vi "SOLAR PLANT MONITORING SYSTEM IN LabVIEW 2.vi"() -> ()   [LabVIEW 2025]
uses:
  <vilib>/Utility/error.llb/DialogType.ctl
  <vilib>/DAQmx/read.llb/DAQmx Read (Analog DBL 1Chan 1Samp).vi
  <vilib>/DAQmx/create/channels.llb/DAQmx Create Channel (AI-Voltage-Basic).vi
  <vilib>/DAQmx/miscellaneous.llb/DAQmx Fill In Error Info.vi
panel:
  in  "custom scale name":tag
  out "I-V curve":cluster{"Y":dbl[], "Y":dbl[]}[](graph)
  out "P-V curve":cluster{"Y":dbl[], "Y":dbl[]}[](graph)
  out "Power curve":dbl(graph)
  out "POWER":dbl(knob) scale=0.0..10.0
  out "Current Chart":dbl(graph)
  out "?":dbl(knob) scale=0.0..10.0
  out "Voltage Chart":dbl(graph)
  out "?":dbl(knob) scale=0.0..50.0
  in  "units":i32(ring)=10348 items=["Volts"=10348, "From Custom Scale"=10065]
  in  "physical channels":tag
  in  "stop":bool
  # "VOLTAGE SENSOR"
  # "CURRENT SENSOR"
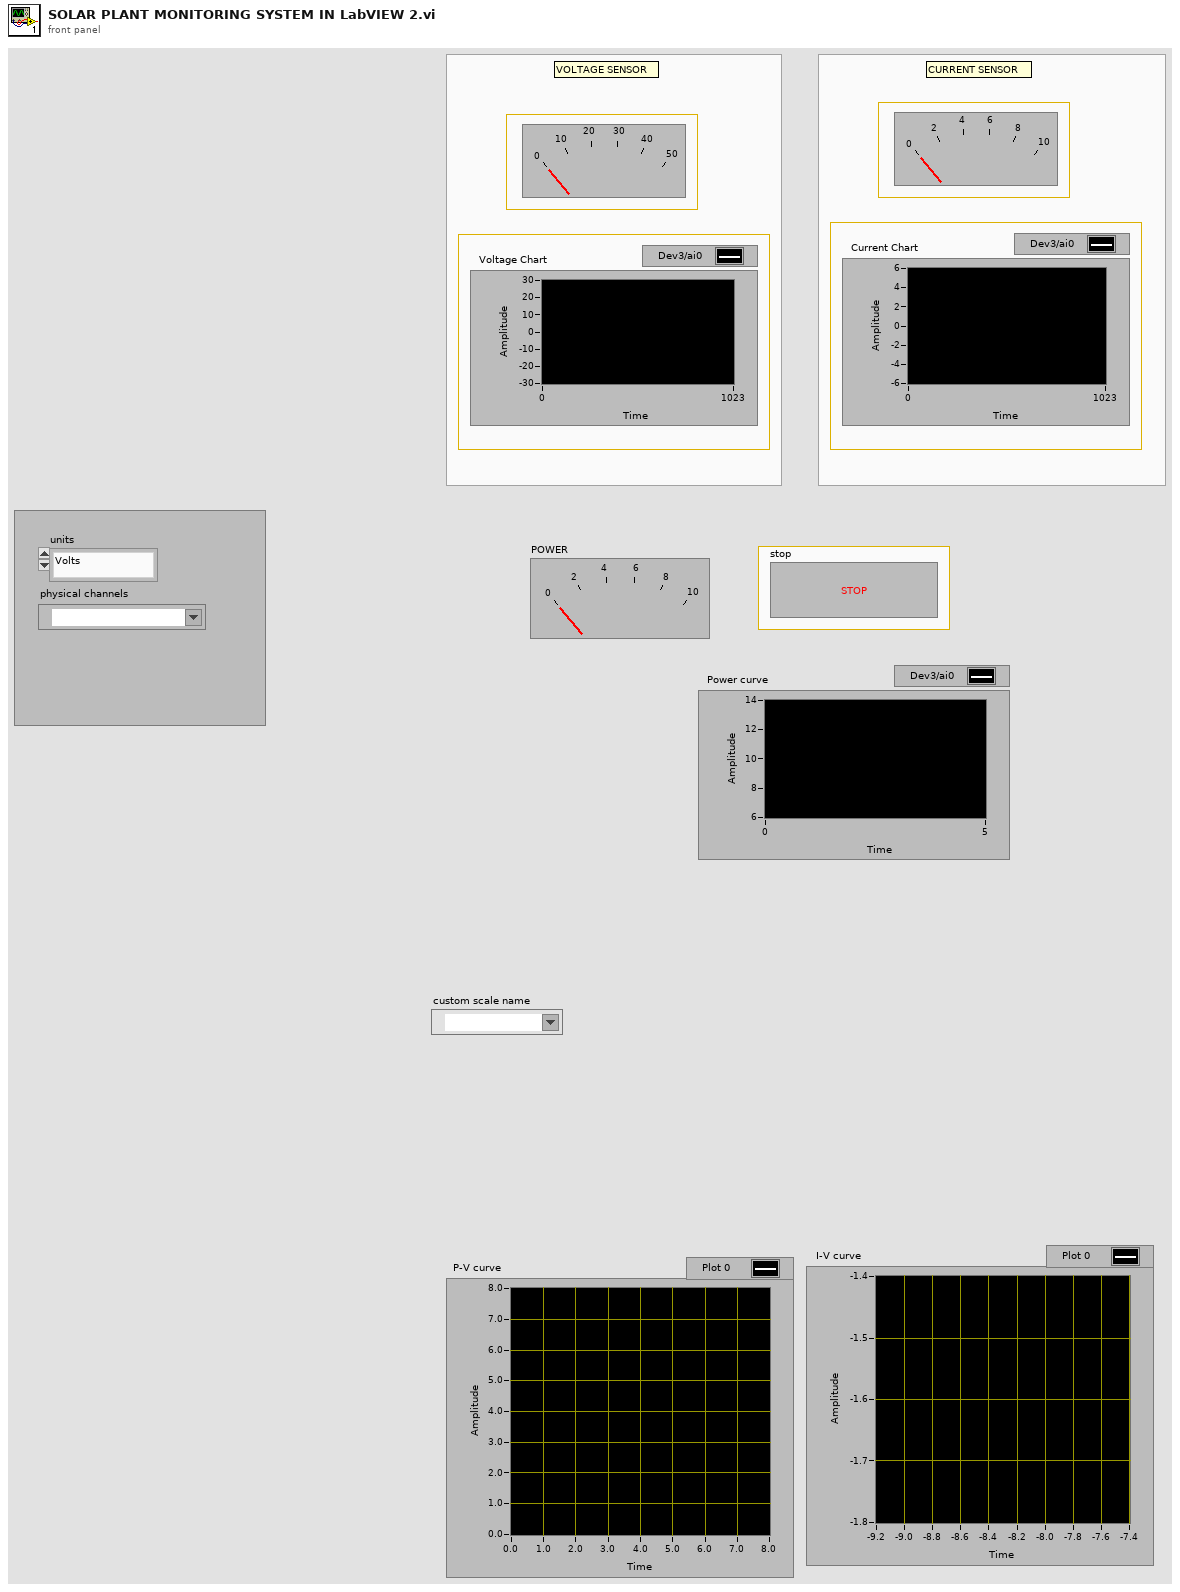
[diagram p1: front panel]
types:
  T1 = typedef "DialogType.ctl" = u16
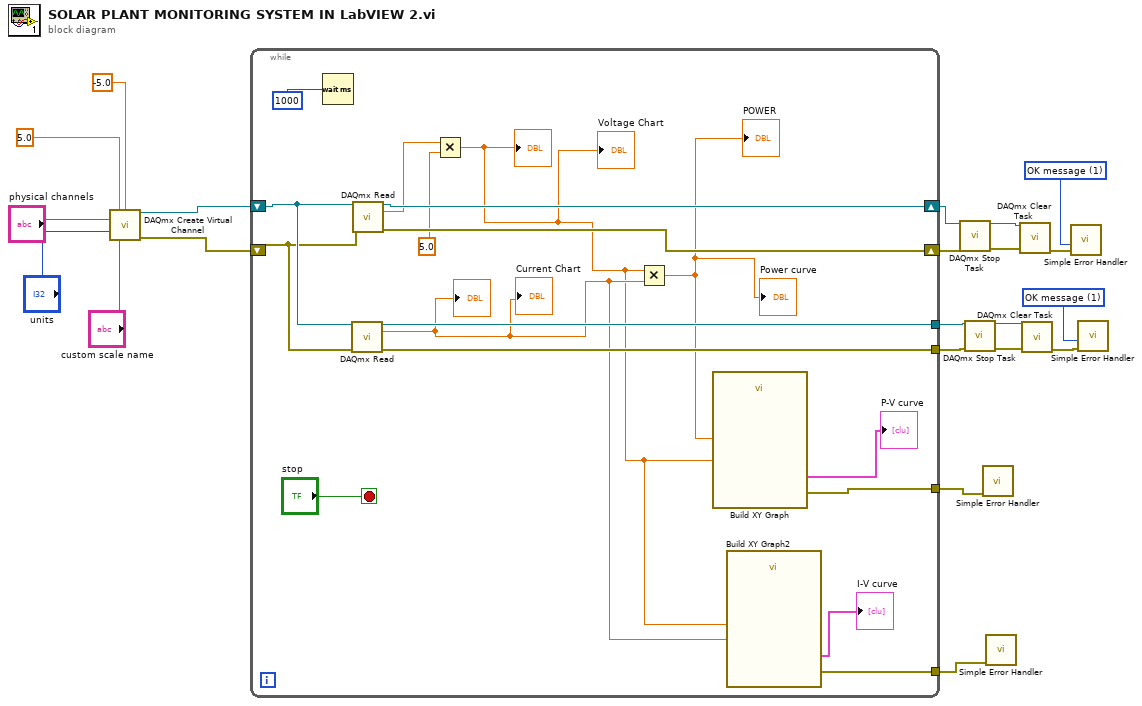
[diagram p0: block diagram]
diagram:
  w8 = T1 1 items=["no dialog", "OK message", "continue or stop message", "OK message + warnings", "continue/stop + warnings"] ("type of dialog (OK msg:1)")
  w12 = T1 1 items=["no dialog", "OK message", "continue or stop message", "OK message + warnings", "continue/stop + warnings"] ("type of dialog (OK msg:1)")
  n1 = call-poly <vilib>:"DAQmx Create Virtual Channel.vi"("maximum value"=5.0, "minimum value"=-5.0, "physical channels"="physical channels", "units"="units", "custom scale name"="custom scale name") -> ("task out"=w19:refnum<k21>, "error out"=w18:errorcluster)  [unwired: 9 in]
  n2 = while {
    shift-right: [w37] -> w16
    shift-left: w19 -> [w33]
    shift-right: [w36] -> w17
    shift-left: w18 -> [w32]
    tunnel: [w31] -> w7
    tunnel: [w30] -> w6
    tunnel: [w27] -> w5
    tunnel: [w22] -> w2
    stop <- "stop" stop-if-true
    n3 = Wait (ms)(milliseconds to wait=u32 1000) -> ()  [unwired: 1 out]
    n4 = call-poly <vilib>:"DAQmx Read.vi"("task/channels in"=w33, "error in"=w32) -> ("task out"=w31:refnum<k21>, "data"=w24:dbl, "error out"=w30:errorcluster)  [unwired: 11 in]
    "?" <- w24
    "Current Chart" <- w24
    n5 = call-poly <vilib>:"DAQmx Read.vi"("task/channels in"=w33, "error in"=w32) -> ("task out"=w37:refnum<k21>, "data"=w35:dbl, "error out"=w36:errorcluster)  [unwired: 11 in]
    n6 = Multiply(x=w35, y=5.0) -> (x*y=w23:dbl)
    "?" <- w23
    "Voltage Chart" <- w23
    n7 = Multiply(x=w23, y=w24) -> (x*y=w28:dbl)
    "POWER" <- w28
    "Power curve" <- w28
    n8 = call "Build XY Graph"("Y Input"=w23, "X Input"=w28) -> ("error out"=w27:errorcluster, "XY Graph"=→"P-V curve":cluster{"X":dbl[], "Y":dbl[]}[])  [unwired: 8 in]
    n9 = call "Build XY Graph2"("Y Input"=w24, "X Input"=w23) -> ("error out"=w22:errorcluster, "XY Graph"=→"I-V curve":cluster{"X":dbl[], "Y":dbl[]}[])  [unwired: 8 in]
  }
  n10 = call <vilib>:"DAQmx Stop Task.vi"("task/channels in"=w16, "error in"=w17) -> ("task out"=w15:refnum<k21>, "error out"=w14:errorcluster)  [unwired: 12 in]
  n11 = call <vilib>:"DAQmx Stop Task.vi"("task/channels in"=w7, "error in"=w6) -> ("task out"=w11:refnum<k21>, "error out"=w10:errorcluster)  [unwired: 12 in]
  n12 = call <vilib>:"Simple Error Handler.vi"("error in (no error)"=w5) -> ()  [unwired: 4 in, 5 out]
  n13 = call <vilib>:"Simple Error Handler.vi"("error in (no error)"=w2) -> ()  [unwired: 4 in, 5 out]
  n14 = call <vilib>:"DAQmx Clear Task.vi"("task in"=w15, "error in"=w14) -> ("error out"=w13:errorcluster)  [unwired: 13 in]
  n15 = call <vilib>:"DAQmx Clear Task.vi"("task in"=w11, "error in"=w10) -> ("error out"=w9:errorcluster)  [unwired: 13 in]
  n16 = call <vilib>:"Simple Error Handler.vi"("type of dialog (OK msg:1)"=w12, "error in (no error)"=w13) -> ()  [unwired: 3 in, 5 out]
  n17 = call <vilib>:"Simple Error Handler.vi"("type of dialog (OK msg:1)"=w8, "error in (no error)"=w9) -> ()  [unwired: 3 in, 5 out]
